vi "0x56_Freeing_data_from_a_prepared_table_parameter.vi"(8 "error in":errorcluster, 10 "Param":cluster{"Номер табличного параметра":i32}, 11 "ParamIn":T1={"ReadIntParam"=TRUE, "ReadDescrParam"=FALSE, "ReadFloatParam"=TRUE, "debug"=FALSE, "ReadJSON"=TRUE, "IP_address"="192.168.1.216", "N_attempts"=3, "type_con"=enum."TCP", "MB_address"=1, "VISA"="COM1", "connection ID"=refnum, "nameDevices"="", "timeout"=0, "port"=0, "type_version"="0F0C0001", "baud_rate"=115200, "VersionControl"=TRUE, "TCP_conn"=TRUE, "WindowSize"=700}) -> (0 "error out":errorcluster, 2 "Ответ":string, 3 "ParamOut":T1={"ReadIntParam"=TRUE, "ReadDescrParam"=FALSE, "ReadFloatParam"=TRUE, "debug"=FALSE, "ReadJSON"=TRUE, "IP_address"="192.168.1.216", "N_attempts"=3, "type_con"=enum."TCP", "MB_address"=1, "VISA"="COM1", "connection ID"=refnum, "nameDevices"="", "timeout"=0, "port"=0, "type_version"="0F0C0001", "baud_rate"=115200, "VersionControl"=TRUE, "TCP_conn"=TRUE, "WindowSize"=700}, 5 "Сообщение об ошибке":bool)   [LabVIEW 2017, in "LV_Unicorn.lvlib"]
uses:
  LV_Unicorn.lvlib
  Control/unicorn_conn.ctl
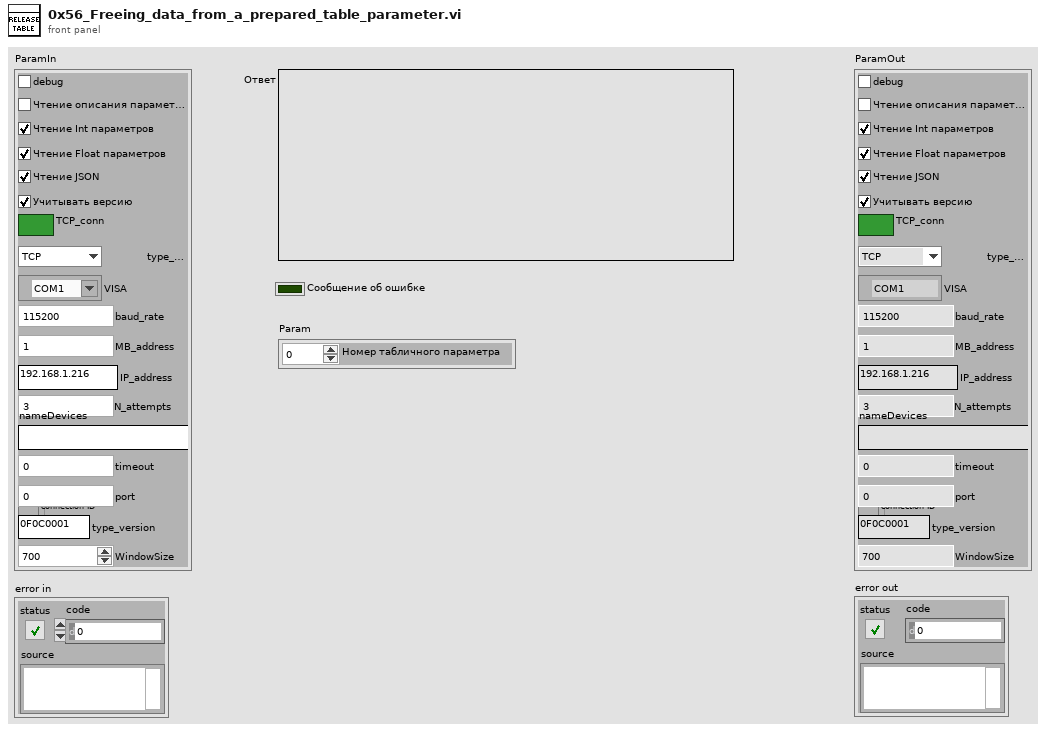
[diagram p1: front panel]
types:
  T1 = typedef "LV_Unicorn.lvlib/unicorn_conn.ctl" = cluster{"ReadIntParam":bool, "ReadDescrParam":bool, "ReadFloatParam":bool, "debug":bool, "ReadJSON":bool, "IP_address":string, "N_attempts":i32, "type_con":enum16{"Serial", "TCP"}, "MB_address":i32, "VISA":refnum<visa-resource-name>, "connection ID":refnum<k5>, "nameDevices":string, "timeout":i32, "port":u16, "type_version":string, "baud_rate":u32, "VersionControl":bool, "TCP_conn":bool, "WindowSize":i32}
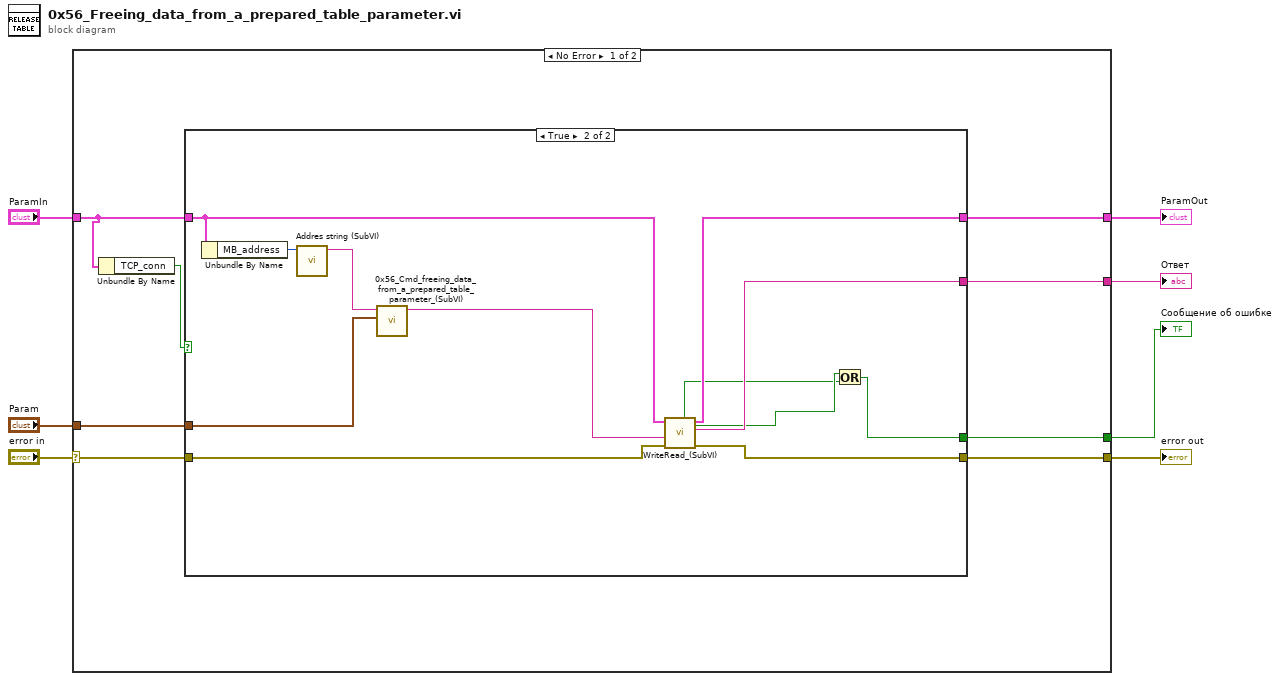
[diagram p0: block diagram]
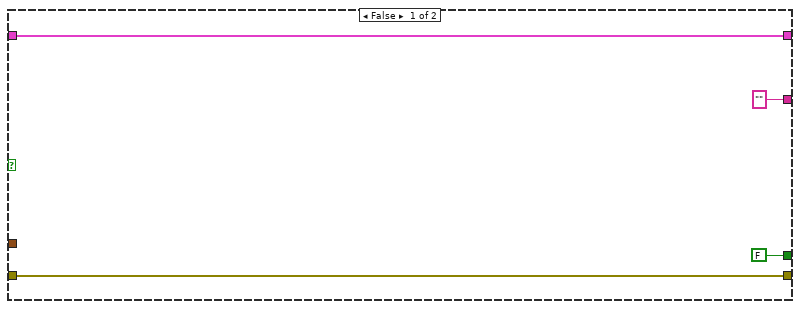
[diagram p2: hidden frame]
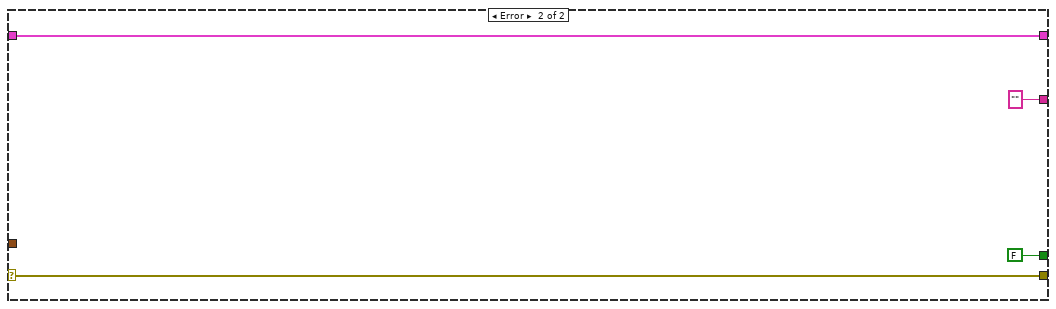
[diagram p3: hidden frame]
diagram:
  n1 = case shown="No Error" "error in" {
    selector: "error in" -> [w13 w34]
    tunnel: "ParamIn" -> [w9 w35]
    tunnel: [w15 w35] -> w6
    tunnel: [w14 w34] -> w5
    tunnel: "Param" -> [w12 _]
    tunnel: [w11 "" ("Ответ")] -> w2
    tunnel: [w10 FALSE ("Сообщение об ошибке")] -> w1
    frame No Error {
      n2 = Unbundle By Name(w9) -> ("TCP_conn"=w8:bool)
      n3 = case shown="True" w8 {
        tunnel: [w19 w31] -> w15
        tunnel: [w16 w30] -> w14
        tunnel: w13 -> [w16 w29]
        tunnel: w9 -> [w19 w28]
        tunnel: w12 -> [_ w24]
        tunnel: ["" ("Ответ") w23] -> w11
        tunnel: [FALSE ("Сообщение об ошибке") w20] -> w10
        frame False {
        }
        frame True {
          n4 = Unbundle By Name(w28) -> ("MB_address"=w27:i32)
          n5 = call "Addres string (SubVI).vi"("Адрес"=w27) -> ("String"=w26:string)  [unwired: 10 in]
          n6 = call "0x56_Cmd_freeing_data_from_a_prepared_table_parameter_(SubVI).vi"("Parameters"=w24, "String in"=w26) -> ("String out"=w25:string)  [unwired: 9 in]
          n7 = call "WriteRead_(SubVI).vi"("error in"=w29, "Запрос"=w25, "ParamIn"=w28) -> ("error out"=w30:errorcluster, "Ответ"=w23:string, "ParamOut"=w31:T1, "ErrorMessage"=w21:bool, "GatewayTimeout"=w22:bool)  [unwired: 4 in]
          n8 = Or(x=w22, y=w21) -> (x .or. y?=w20:bool)
        }
      }
    }
    frame Error {
    }
  }
  "error out" <- w5
  "ParamOut" <- w6
  "Ответ" <- w2
  "Сообщение об ошибке" <- w1
